vi "fg_installer_location.vi"(7 "fg_command":T1=enum."read", 8 "error in (no error)":errorcluster, 11 "path [] in":path[](array[path])) -> (0 "error out":errorcluster, 3 "path [] out":path[](array[path]))   [LabVIEW 2015, in "lv-post-installer.lvlib"]
uses:
  lv-post-installer.lvlib
  _controls/fg_command.ctl
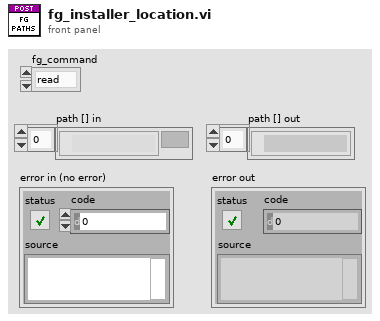
[diagram p1: front panel]
types:
  T1 = typedef "lv-post-installer.lvlib/fg_command.ctl" = enum16{"null", "initialize", "read", "write", "shutdown"}
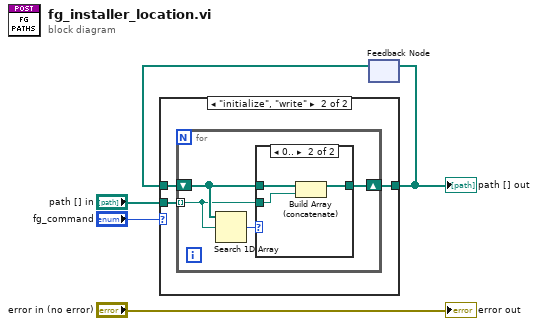
[diagram p0: block diagram]
diagram:
  n1 = feedback #1() -> (w3:path[])  [unwired: 1 in]
  n2 = case shown="\"initialize\", \"write\"" "fg_command" {
    tunnel: "path [] in" -> [_ w7]
    tunnel: [w6 w8] -> w2
    tunnel: w3 -> [w6 w9]
    frame Default {
    }
    frame "initialize", "write" {
      n3 = for {
        shift-right: [w11] -> w8
        shift-left: w9 -> [w13]
        tunnel: w7 -> [w10] mode=indexing
        n4 = Search 1D Array(1D array=w13, element=w10) -> (index of element=w12:i32)  [unwired: 1 in]
        n5 = case shown="0.." w12 {
          tunnel: w13 -> [w14 w17]
          tunnel: w10 -> [_ w16]
          tunnel: [w14 w15] -> w11
          frame Default {
          }
          frame 0.. {
            n6 = Build Array (concatenate)(w17, w16) -> (w15:path[])
          }
        }
      }
    }
  }
  "path [] out" <- w2
  n7 = feedback-in #1(w2) -> ()
  "error out" <- "error in (no error)"
